vi "_Calibrate Fast DAC.vi"(1 "Mass (100x)":i32, 2 "Address":u16) -> (0 "DAC":u32)   [LabVIEW 2015]
uses:
  <vilib>/rvi/Memory/Memory_Emulation/nirvimemoryEmulation.vi
  <vilib>/rvi/Memory/Memory_Emulation/nirvimemoryFastEmulation.vi
  <vilib>/rvi/DataTransferAndStorage/Container/Common/niFpgaContainerGetUniqueNameForEmu.vi
  <vilib>/rvi/Memory/Memory_Emulation/niFpgaMemoryEmulationCacheClearOnFirstRun.vi
  <vilib>/rvi/Memory/Memory_Emulation/nirvimemoryEmulationManagerCache_MakeExclusive.vi
  <vilib>/rvi/Memory/Memory_Emulation/niFpgaMemoryEmulationValidateCache.vi
  <vilib>/rvi/Memory/Memory_Emulation/nirvimemoryEmulationManagerCache_InsertValue.vi
  <vilib>/Utility/error.llb/Clear Errors.vi
  <vilib>/rvi/Memory/Memory_Emulation/nirvimemoryEmulationManagerCache_ReleaseExclusive.vi
  <vilib>/rvi/Memory/Memory_Emulation/nirvimemoryEmulationManagerCache_GetValue.vi
  <vilib>/rvi/Emulation/niFpgaEmulationIsFPGAContextNoSignature.vi
  <vilib>/rvi/Emulation/niFpgaSctlEmulationGetInTimedLoop.vi
  <vilib>/rvi/Memory/Memory_Emulation/nirvimemoryEmulationManagerCache_SetValue.vi
  <vilib>/rvi/Emulation/niFpgaSctlEmulationResourceMgr.vi
  <vilib>/rvi/DataTransferAndStorage/Container/XNode/niFpgaContainer.xnode
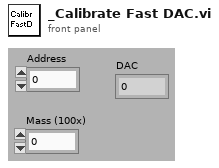
[diagram p1: front panel]
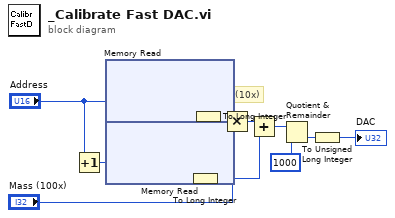
[diagram p0: block diagram]
diagram:
  # "offset"
  # "slope (10x)"
  n1 = Increment(x="Address") -> (x+1=w6:u16)
  n2 = xnode ("Memory Read")("Address"="Address") -> ("Data"=w7:u32)  [unwired: 1 in, 1 out]
  n3 = xnode ("Memory Read")("Address"=w6) -> ("Data"=w10:u32)  [unwired: 1 in, 1 out]
  n4 = To Long Integer(number=w10) -> (32bit integer=w12:i32)
  n5 = To Long Integer(number=w7) -> (32bit integer=w11:i32)
  n6 = Multiply(x=w11, y="Mass (100x)") -> (x*y=w9:i32)
  n7 = Add(x=w9, y=w12) -> (x+y=w3:i32)
  n8 = Quotient & Remainder(x=w3, y=1000) -> (floor(x/y)=w1:i32)  [unwired: 1 out]
  n9 = To Unsigned Long Integer(number=w1) -> (unsigned 32bit integer=→"DAC":u32)
